vi "Write_metadata_subVI_BM.vi"(6 "Analyte":string, 8 "Analysis Type":T3(ring), 9 "Mode Selection":T2(ring), 10 "sample volume":dbl=10.0, 11 "Metadata":T1={"Local save location:"="C:\\Users\\LabPC1\\OneDrive\\Desktop\\OSSCAR_metadata\\Test_metadata", "Cruise ID"="LaPerouse", "Sampling Timestamp"="2023-07-19 15:23:13", "Elution Timestamp"="2023-07-19 15:29:12", "GPS_Latitude"=-999.0, "GPS_Longitude"=-999.0, "DMS_std_conc"=0.0, "DMSP_std_conc"=0.0, "DMSO_std_conc"=0.0, "Std_index"=0.0, "Initial Trap Temp (oC)"=174.0, "Max Trap Temp (oC)"=174.0, "Final Trap Temp (oC)"=0.0, "Flow Rate (mL/min)"=0.0, "Comment"="", "GPS_Minute"=-999.0, "GPS_Day"=-999.0, "GPS_jd"=-999.0, "GPS_Hour"=-999.0, "GPS_Second"=-999.0, "GPS Baud"=4800.0, "COM Port (GPS)"="COM10", "Use GPS?"=FALSE, "Format Date"="%d-%d-%d"} {"GPS_Latitude" format="%_4g"; "GPS_Longitude" format="%_4g"; "GPS_jd" format="%_5g"; "Std_index" format="%.2g"; "DMSO_std_conc" format="%.2f"; "DMSP_std_conc" format="%.2f"; "DMS_std_conc" format="%.2f"}) -> ()   [LabVIEW 2021]
uses:
  <vilib>/Utility/file.llb/Write Delimited Spreadsheet (string).vi
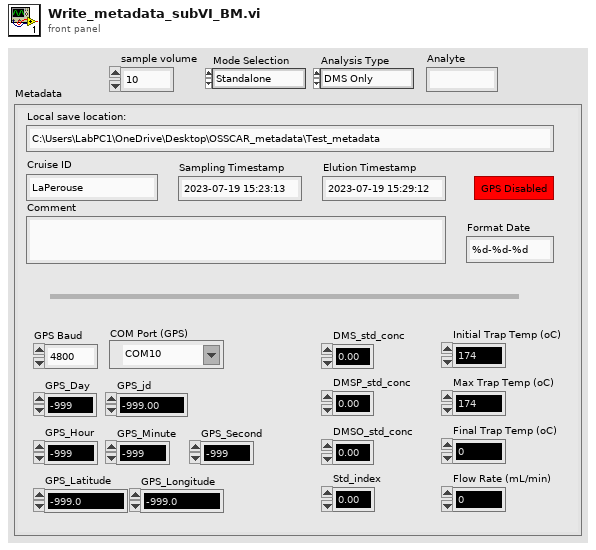
[diagram p1: front panel]
types:
  T1 = cluster{"Local save location:":string, "Cruise ID":string, "Sampling Timestamp":string, "Elution Timestamp":string, "GPS_Latitude":dbl, "GPS_Longitude":dbl, "DMS_std_conc":dbl, "DMSP_std_conc":dbl, "DMSO_std_conc":dbl, "Std_index":dbl, "Initial Trap Temp (oC)":dbl, "Max Trap Temp (oC)":dbl, "Final Trap Temp (oC)":dbl, "Flow Rate (mL/min)":dbl, "Comment":string, "GPS_Minute":dbl, "GPS_Day":dbl, "GPS_jd":dbl, "GPS_Hour":dbl, "GPS_Second":dbl, "GPS Baud":dbl, "COM Port (GPS)":refnum<visa-resource-name>, "Use GPS?":bool, "Format Date":string}
  T2 = enum16{"Standalone", "Analysis", "Standard Curve", "Point Std"}
  T3 = enum16{"DMS Only", "DMS/O", "DMS/P", "DMS/O/P", "DMSO Only"}
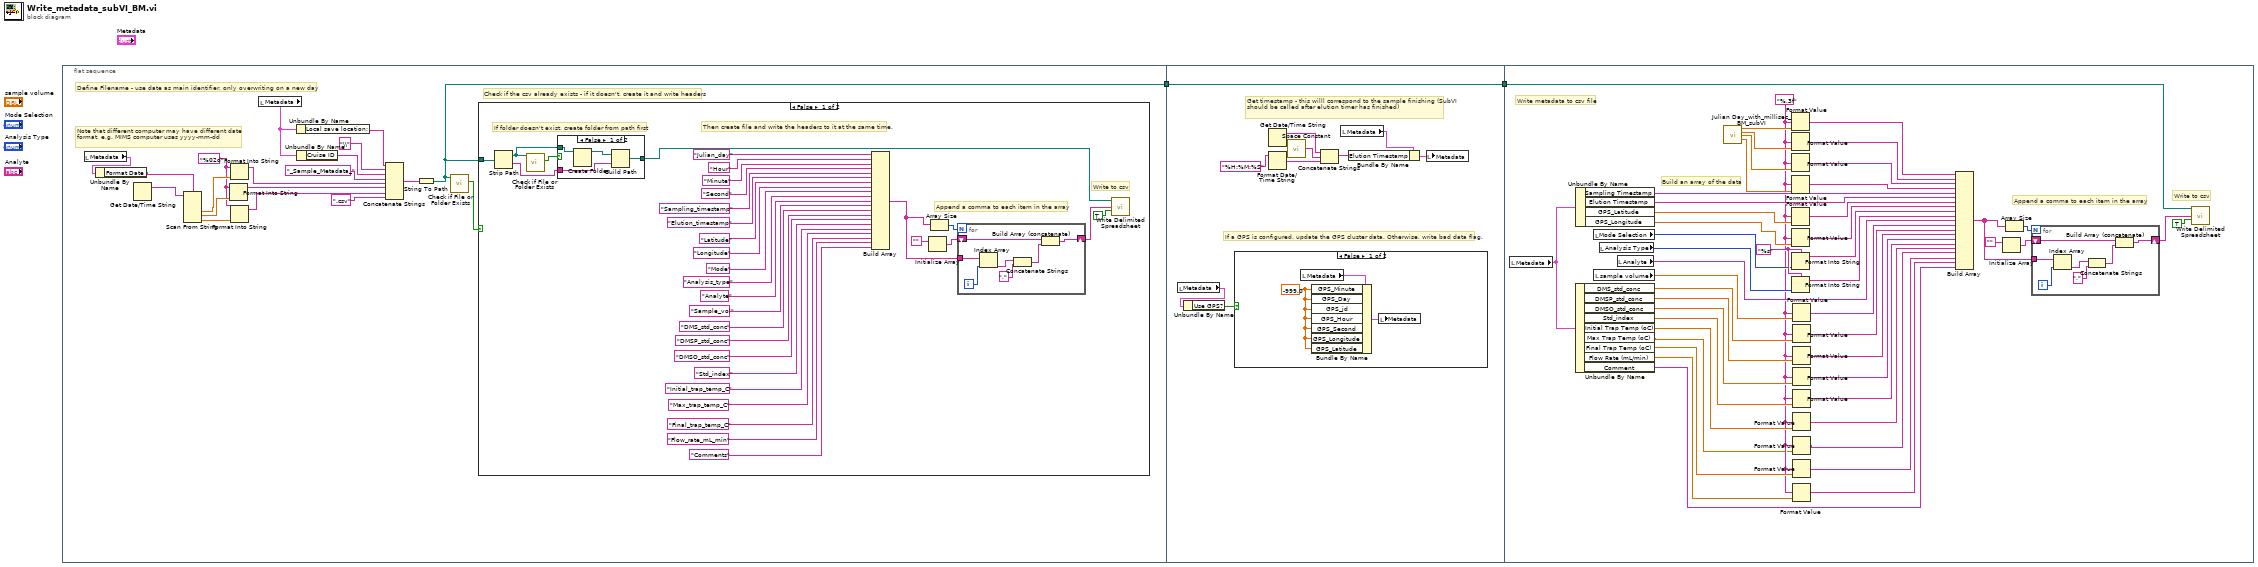
[diagram p0: block diagram]
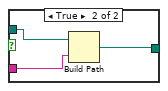
[diagram p2: hidden frame]
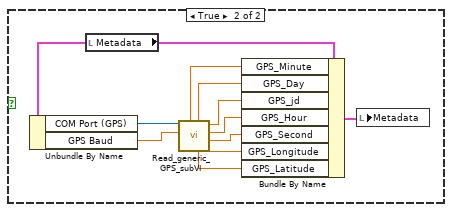
[diagram p4: hidden frame]
diagram:
  n1 = flat-sequence {
    tunnel: [w3] -> w2
    tunnel: [w70] -> w1
    tunnel: w2 -> [w70]
    tunnel: w1 -> [w112]
    frame #0 {
      w16 = "%02d"
      # "Check if the csv already exists - if it doesn't, create it and write headers"
      # "Define Filename - use date as main identifier, only overwriting on a new day"
      # "Note that different computer may have different date format, e.g. MIMS computer uses yyyy-mm-dd"
      n2 = local read "Metadata"() -> (w5:T1)
      n3 = Unbundle By Name(w5) -> ("Format Date"=w4:string)
      n4 = Get Date/Time String() -> (date string=w17:string)  [unwired: 3 in, 1 out]
      n5 = Scan From String(format string=w4, input string=w17) -> (output 1=w19:dbl, output 2=w20:dbl, output 3=w21:dbl)  [unwired: 5 in, 3 out]
      n6 = Format Into String(format string=w16, w20) -> (resulting string=w10:string)  [unwired: 2 in, 1 out]
      n7 = Format Into String(format string=w16, w19) -> (resulting string=w11:string)  [unwired: 2 in, 1 out]
      n8 = Format Into String(format string=w16, w21) -> (resulting string=w18:string)  [unwired: 2 in, 1 out]
      n9 = local read "Metadata"() -> (w7:T1)
      n10 = Unbundle By Name(w7) -> ("Local save location:"=w9:string)
      n11 = Unbundle By Name(w7) -> ("Cruise ID"=w8:string)
      n12 = Concatenate Strings(w9, "\\", w8, "_Sample_Metadata_", w11, w10, w18, ".csv") -> (w13:string)
      n13 = String To Path(string=w13) -> (path=w3:path)
      n14 = call <vilib>:"Check if File or Folder Exists.vi"("path"=w3) -> ("file or folder exists?"=w6:bool)  [unwired: 8 in, 2 out]
      n15 = case shown="False" w6 {
        tunnel: w3 -> [w35 _]
        frame False {
          # "Write to csv"
          # "Append a comma to each item in the array"
          # "If folder doesn't exist, create folder from path first"
          # "Then create file and write the headers to it at the same time."
          n16 = Strip Path(path=w35) -> (stripped path=w33:path, name=w32:string)
          n17 = call <vilib>:"Check if File or Folder Exists.vi"("path"=w33) -> ("file or folder exists?"=w34:bool)  [unwired: 8 in, 2 out]
          n18 = case shown="False" w34 {
            tunnel: w33 -> [w64 w67]
            tunnel: w32 -> [w62 w66]
            tunnel: [w61 w65] -> w31
            frame False {
              n19 = Create Folder(path (use dialog)=w64) -> (created path=w63:path)  [unwired: 2 in, 2 out]
              n20 = Build Path(base path=w63, name or relative path=w62) -> (appended path=w61:path)
            }
            frame True {
              n21 = Build Path(base path=w67, name or relative path=w66) -> (appended path=w65:path)
            }
          }
          n22 = Build Array("Julian_day" ("string"), "Hour" ("string 2"), "Minute" ("string 3"), "Second" ("string 4"), "Sampling_timestamp" ("string 4"), "Elution_timestamp" ("string 4"), "Latitude" ("string 4"), "Longitude" ("string 4"), "Mode" ("string 4"), "Analysis_type" ("string 4"), "Analyte" ("string 4"), "Sample_vol" ("string 4"), "DMS_std_conc" ("string 4"), "DMSP_std_conc" ("string 4"), "DMSO_std_conc" ("string 4"), "Std_index" ("string 4"), "Initial_trap_temp_C" ("string 4"), "Max_trap_temp_C" ("string 4"), "Final_trap_temp_C" ("string 4"), "Flow_rate_mL_min" ("string 4"), "Comments" ("string 4")) -> (w26:string[])
          n23 = Initialize Array("") -> (w28:string[])  [unwired: 1 in]
          n24 = Array Size(array=w26) -> (size(s)=w29:i32)
          n25 = for {
            N: w29 -> [_]
            shift-right: [w56] -> w25
            shift-left: w28 -> [w55]
            tunnel: w26 -> [w54]
            i -> [w60]
            n26 = Index Array(array=w54, index=w60) -> (element=w58:string)
            n27 = Concatenate Strings(w58, "," ("string")) -> (w57:string)
            n28 = Build Array (concatenate)(w55, w57) -> (w56:string[])
          }
          n29 = call-poly <vilib>:"Write Delimited Spreadsheet.vi"("file path (dialog if empty)"=w31, "1D data"=w25, "append to file? (new file:F)"=TRUE) -> ()  [unwired: 11 in, 2 out]
        }
        frame True {
          # "If file (and folder) exists, do nothing here - headers already exist, so append the new data in the next few frames"
        }
      }
    }
    frame #1 {
      # "If a GPS is configured, update the GPS cluster data. Otherwise, write bad data flag."
      # "Get timestamp - this willl correspond to the sample finishing (SubVI should be called after elution timer has finished)"
      n30 = local read "Metadata"() -> (w69:T1)
      n31 = Unbundle By Name(w69) -> ("Use GPS?"=w68:bool)
      n32 = case shown="False" w68 {
        frame False {
          w78 = -999.0 ("GPS_Minute")
          n33 = local read "Metadata"() -> (w79:T1)
          n34 = Bundle By Name(cluster=w79, "GPS_Minute"=w78, "GPS_Day"=w78, "GPS_jd"=w78, "GPS_Hour"=w78, "GPS_Second"=w78, "GPS_Longitude"=w78, "GPS_Latitude"=w78) -> (w80:T1)
          n35 = local write "Metadata"(w80) -> ()
        }
        frame True {
          n36 = local read "Metadata"() -> (w83:T1)
          n37 = Unbundle By Name(w83) -> ("COM Port (GPS)"=w81:refnum<visa-resource-name>, "GPS Baud"=w82:dbl)
          n38 = call "Read_generic_GPS_subVI.vi"("Baud Rate"=w82, "VISA resource name"=w81) -> ("Longitude W"=w89:dbl, "GPS\nSeconds"=w88:dbl, "GPS\nHour"=w87:dbl, "GPS JD"=w86:dbl, "Latitude N"=w90:dbl, "GPS\nDay"=w85:dbl, "GPS\nMinute"=w84:dbl)  [unwired: 3 in]
          n39 = Bundle By Name(cluster=w83, "GPS_Minute"=w84, "GPS_Day"=w85, "GPS_jd"=w86, "GPS_Hour"=w87, "GPS_Second"=w88, "GPS_Longitude"=w89, "GPS_Latitude"=w90) -> (w91:T1)
          n40 = local write "Metadata"(w91) -> ()
        }
      }
      n41 = Get Date/Time String() -> (date string=w74:string)  [unwired: 3 in, 1 out]
      n42 = Format Date/Time String(time format string (%c)="%H:%M:%S" ("format string")) -> (date/time string=w73:string)  [unwired: 2 in]
      n43 = call <vilib>:"Space Constant.vi"() -> ("String"=w72:string)
      n44 = Concatenate Strings(w74, w72, w73) -> (w76:string)
      n45 = local read "Metadata"() -> (w75:T1)
      n46 = Bundle By Name(cluster=w75, "Elution Timestamp"=w76) -> (w77:T1)
      n47 = local write "Metadata"(w77) -> ()
    }
    frame #2 {
      w99 = "%s" ("format string")
      w94 = "%.3f"
      # "Build an array of the data"
      # "Write to csv"
      # "Append a comma to each item in the array"
      # "Write metadata to csv file"
      n48 = local read "Metadata"() -> (w100:T1)
      n49 = Unbundle By Name(w100) -> ("DMS_std_conc"=w120:dbl, "DMSP_std_conc"=w121:dbl, "DMSO_std_conc"=w122:dbl, "Std_index"=w123:dbl, "Initial Trap Temp (oC)"=w124:dbl, "Max Trap Temp (oC)"=w93:dbl, "Final Trap Temp (oC)"=w125:dbl, "Flow Rate (mL/min)"=w126:dbl, "Comment"=w139:string)
      n50 = Unbundle By Name(w100) -> ("Sampling Timestamp"=w105:string, "Elution Timestamp"=w104:string, "GPS_Latitude"=w103:dbl, "GPS_Longitude"=w102:dbl)
      n51 = local read "Mode Selection"() -> (w96:T2)
      n52 = local read "sample volume"() -> (w101:dbl)
      n53 = local read "Analysis Type"() -> (w97:T3)
      n54 = local read "Analyte"() -> (w95:string)
      n55 = call "Julian Day_with_millisec_BM_subVI.vi"() -> ("Julian Day"=w135:dbl, "hour"=w136:dbl, "minute"=w137:dbl, "Decimal second"=w138:dbl)  [unwired: 11 in, 1 out]
      n56 = Format Value(format string=w94, value (0)=w135) -> (output string=w113:string)  [unwired: 1 in]
      n57 = Format Value(format string=w94, value (0)=w136) -> (output string=w114:string)  [unwired: 1 in]
      n58 = Format Value(format string=w94, value (0)=w137) -> (output string=w115:string)  [unwired: 1 in]
      n59 = Format Value(format string=w94, value (0)=w138) -> (output string=w116:string)  [unwired: 1 in]
      n60 = Format Value(format string=w94, value (0)=w103) -> (output string=w117:string)  [unwired: 1 in]
      n61 = Format Value(format string=w94, value (0)=w102) -> (output string=w118:string)  [unwired: 1 in]
      n62 = Format Into String(format string=w99, w96) -> (resulting string=w119:string)  [unwired: 2 in, 1 out]
      n63 = Format Into String(format string=w99, w97) -> (resulting string=w98:string)  [unwired: 2 in, 1 out]
      n64 = Format Value(format string=w94, value (0)=w101) -> (output string=w127:string)  [unwired: 1 in]
      n65 = Format Value(format string=w94, value (0)=w120) -> (output string=w128:string)  [unwired: 1 in]
      n66 = Format Value(format string=w94, value (0)=w121) -> (output string=w129:string)  [unwired: 1 in]
      n67 = Format Value(format string=w94, value (0)=w122) -> (output string=w130:string)  [unwired: 1 in]
      n68 = Format Value(format string=w94, value (0)=w123) -> (output string=w131:string)  [unwired: 1 in]
      n69 = Format Value(format string=w94, value (0)=w124) -> (output string=w132:string)  [unwired: 1 in]
      n70 = Format Value(format string=w94, value (0)=w93) -> (output string=w92:string)  [unwired: 1 in]
      n71 = Format Value(format string=w94, value (0)=w125) -> (output string=w133:string)  [unwired: 1 in]
      n72 = Format Value(format string=w94, value (0)=w126) -> (output string=w134:string)  [unwired: 1 in]
      n73 = Build Array(w113, w114, w115, w116, w105, w104, w117, w118, w119, w98, w95, w127, w128, w129, w130, w131, w132, w92, w133, w134, w139) -> (w107:string[])
      n74 = Initialize Array("") -> (w109:string[])  [unwired: 1 in]
      n75 = Array Size(array=w107) -> (size(s)=w110:i32)
      n76 = for {
        N: w110 -> [_]
        shift-right: [w142] -> w106
        shift-left: w109 -> [w141]
        tunnel: w107 -> [w140]
        i -> [w146]
        n77 = Index Array(array=w140, index=w146) -> (element=w144:string)
        n78 = Concatenate Strings(w144, "," ("string")) -> (w143:string)
        n79 = Build Array (concatenate)(w141, w143) -> (w142:string[])
      }
      n80 = call-poly <vilib>:"Write Delimited Spreadsheet.vi"("file path (dialog if empty)"=w112, "1D data"=w106, "append to file? (new file:F)"=TRUE) -> ()  [unwired: 11 in, 2 out]
    }
  }
